vi "Write_uTTA_CalibrationFile.vi"(7 "Junction Calibration":T1(array[cluster]), 8 "error in (no error)":errorcluster, 9 "ADC":cluster{"Offset":dbl[], "Gain":dbl[]}, 10 "PGA":cluster{"Offset":dbl[], "Gain":dbl[]}, 11 "selected path":path) -> (0 "error out":errorcluster)   [LabVIEW 2021]
uses:
  <vilib>/Utility/config.llb/Write Key (Double).vi
  <vilib>/Utility/config.llb/NI_LVConfig.lvlib
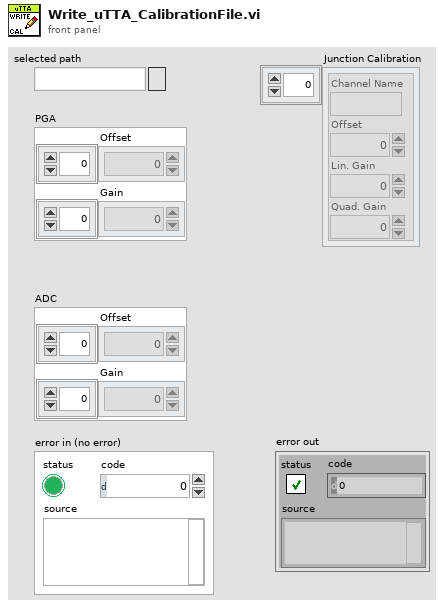
[diagram p1: front panel]
types:
  T1 = cluster{"Channel Name":string, "Offset":dbl, "Lin. Gain":dbl, "Quad. Gain":dbl}[]
  T2 = typedef "NI_LVConfig.lvlib/Config Data RefNum.ctl" = refnum<k1>
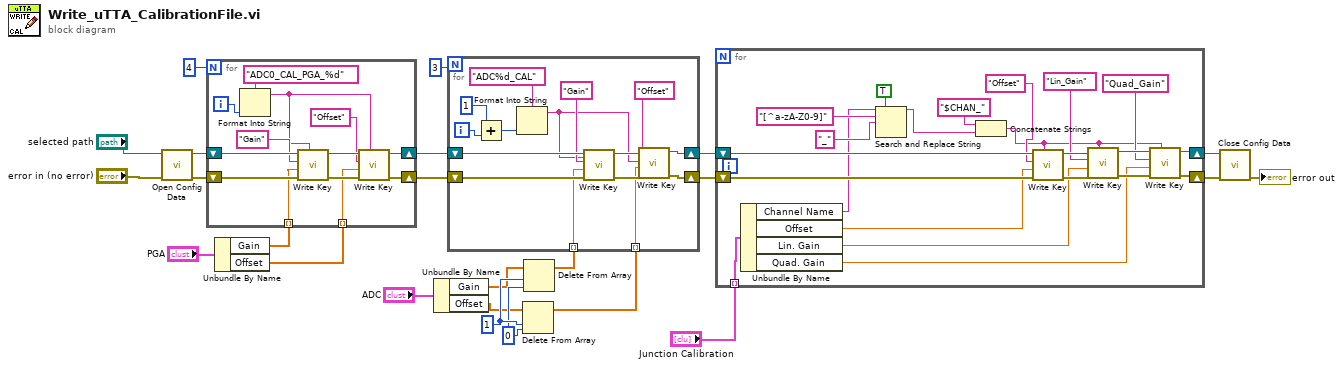
[diagram p0: block diagram]
diagram:
  w13 = 1 ("length")
  w12 = 0 ("index")
  n1 = call <vilib>:"Open Config Data.vi"("error in (no error)"="error in (no error)", "configuration file path"="selected path") -> ("error out"=w19:errorcluster, "refnum"=w18:T2)  [unwired: 7 in, 1 out]
  n2 = Unbundle By Name("PGA") -> ("Gain"=w7:dbl[], "Offset"=w8:dbl[])
  n3 = for {
    N: 4 -> [_]
    shift-right: [w26] -> w3
    shift-left: w18 -> [w35]
    shift-right: [w25] -> w2
    shift-left: w19 -> [w34]
    tunnel: w7 -> [w30] mode=indexing
    tunnel: w8 -> [w29] mode=indexing
    i -> [w36]
    n4 = Format Into String(format string="ADC0_CAL_PGA_%d", w36) -> (resulting string=w28:string)  [unwired: 2 in, 1 out]
    n5 = call-poly <vilib>:"Write Key.vi"("section"=w28, "error in (no error)"=w34, "value"=w30, "key"="Gain", "refnum"=w35) -> ("error out"=w31:errorcluster, "refnum out"=w32:T2)  [unwired: 4 in, 1 out]
    n6 = call-poly <vilib>:"Write Key.vi"("section"=w28, "error in (no error)"=w31, "value"=w29, "key"="Offset", "refnum"=w32) -> ("error out"=w25:errorcluster, "refnum out"=w26:T2)  [unwired: 4 in, 1 out]
  }
  n7 = Unbundle By Name("ADC") -> ("Gain"=w10:dbl[], "Offset"=w11:dbl[])
  n8 = Delete From Array(array=w11, length=w13, index=w12) -> (array with subset deleted=w14:dbl[])  [unwired: 1 out]
  n9 = Delete From Array(array=w10, length=w13, index=w12) -> (array with subset deleted=w15:dbl[])  [unwired: 1 out]
  n10 = for {
    N: 3 -> [_]
    shift-right: [w39] -> w20
    shift-left: w3 -> [w48]
    shift-right: [w38] -> w21
    shift-left: w2 -> [w47]
    tunnel: w14 -> [w40] mode=indexing
    tunnel: w15 -> [w45] mode=indexing
    i -> [w52]
    n11 = Add(x=1, y=w52) -> (x+y=w51:i32)
    n12 = Format Into String(format string="ADC%d_CAL", w51) -> (resulting string=w42:string)  [unwired: 2 in, 1 out]
    n13 = call-poly <vilib>:"Write Key.vi"("section"=w42, "error in (no error)"=w47, "value"=w45, "key"="Gain", "refnum"=w48) -> ("error out"=w44:errorcluster, "refnum out"=w43:T2)  [unwired: 4 in, 1 out]
    n14 = call-poly <vilib>:"Write Key.vi"("section"=w42, "error in (no error)"=w44, "value"=w40, "key"="Offset", "refnum"=w43) -> ("error out"=w38:errorcluster, "refnum out"=w39:T2)  [unwired: 4 in, 1 out]
  }
  n15 = for {
    shift-right: [w64] -> w22
    shift-left: w20 -> [w74]
    shift-right: [w63] -> w23
    shift-left: w21 -> [w73]
    tunnel: "Junction Calibration" -> [w65] mode=indexing
    n16 = Unbundle By Name(w65) -> ("Channel Name"=w54:string, "Offset"=w62:dbl, "Lin. Gain"=w61:dbl, "Quad. Gain"=w60:dbl)
    n17 = Search and Replace String(replace all?=TRUE ("replace all? (F)"), input string=w54, search string="[^a-zA-Z0-9]", replace string="_" ("replace string (\"\")")) -> (result string=w53:string)  [unwired: 4 in, 3 out]
    n18 = Concatenate Strings("$CHAN_" ("string"), w53) -> (w58:string)
    n19 = call-poly <vilib>:"Write Key.vi"("section"=w58, "error in (no error)"=w73, "value"=w62, "key"="Offset", "refnum"=w74) -> ("error out"=w71:errorcluster, "refnum out"=w70:T2)  [unwired: 4 in, 1 out]
    n20 = call-poly <vilib>:"Write Key.vi"("section"=w58, "error in (no error)"=w71, "value"=w61, "key"="Lin_Gain", "refnum"=w70) -> ("error out"=w67:errorcluster, "refnum out"=w68:T2)  [unwired: 4 in, 1 out]
    n21 = call-poly <vilib>:"Write Key.vi"("section"=w58, "error in (no error)"=w67, "value"=w60, "key"="Quad_Gain", "refnum"=w68) -> ("error out"=w63:errorcluster, "refnum out"=w64:T2)  [unwired: 4 in, 1 out]
  }
  n22 = call <vilib>:"Close Config Data.vi"("error in (no error)"=w23, "refnum"=w22) -> ("error out"=→"error out":errorcluster)  [unwired: 8 in, 1 out]
